vi "NoParent_DefaultValuesSet.vi"() -> (0 "error out":errorcluster)   [LabVIEW 2019, in "ResultTreeTest.lvlib" / "AddTestCase.lvlib"]
uses:
  AddTestCase.lvlib
  f803b9a4-b9bb-4b95-b977-91ac30d3708d.vi
  Constraint/IsEqual/Create.vi
  Constraint/IsEqual/IsEqual.lvclass
  ResultTree/ResultTree.lvclass
panel:
  in  "Tree":string(tree)
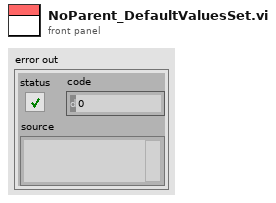
[diagram p1: front panel]
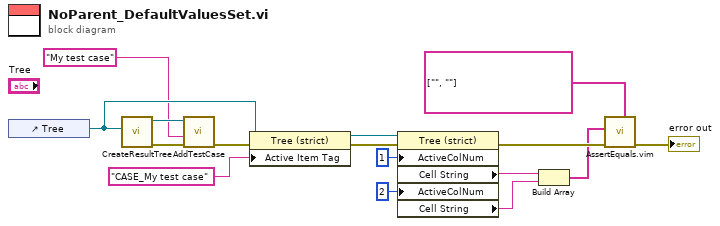
[diagram p0: block diagram]
diagram:
  n1 = control-ref of="Tree"() -> (w15:refnum<vi>)
  n2 = call "CreateResultTree.vi"("Tree Refnum"=w15) -> ("error out"=w14:errorcluster, "ResultTree out"=w12:refnum<class "ResultTree.lvclass">)  [unwired: 9 in]
  n3 = call "AddTestCase.vi"("error in (no error)"=w14, "Name"="My test case", "ResultTree in"=w12) -> ("error out"=w13:errorcluster)  [unwired: 7 in, 1 out]
  n4 = property class="Tree (strict)"(reference=w15, error in=w13, "Active Item Tag"="CASE_My test case" ("Active Item:Tag")) -> (reference out=w8:refnum<vi>, error out=w11:errorcluster)
  n5 = property class="Tree (strict)"(reference=w8, error in=w11, "ActiveColNum"=1 ("Active Cell:Active Column Number"), "ActiveColNum"=2 ("Active Cell:Active Column Number")) -> (error out=w9:errorcluster, "Cell String"=w5:string, "Cell String"=w4:string)  [unwired: 1 out]
  n6 = Build Array(w5, w4) -> (w3:string[])
  n7 = call "AssertEquals.vim"("Expected"=string[] ["", ""] ("All Tags"), "error in (no error)"=w9, "Actual"=w3) -> ("error out"=→"error out":errorcluster)  [unwired: 8 in]
